vi "Send Alternative Long Execution Method.vi"(7 "Async Message Settings":T1={"Message Priority (Normal)"=enum."Normal", "Async Call Method (Call and Collect)"=enum."Call and Collect", "VI Refnum Lifetime (Destroy on Actor Exit)"=enum."Destroy on Actor Exit", "Report Errors (T)"=TRUE, "Caller Enqueuer"=refnum, "Completion Notification Msg"=refnum}, 8 "error in (no error)":errorcluster, 11 "Message Enqueuer in":refnum<class "Message Enqueuer.lvclass">) -> (0 "error out":errorcluster, 2 "GUID":string, 3 "Message Enqueuer out":refnum<class "Message Enqueuer.lvclass">)   [LabVIEW 2023, in "Async Methods Actor Example.lvlib" / "Alternative Long Execution Method Msg.lvclass"]
doc: "Sends the <b>Async Methods Actor Example.lvlib:Alternative Long Execution Method Msg.lvclass</b> Async Message.\n\nThis message will call <b>Alternative Long Execution Method.vi</b> on the <b>Async Methods Actor Example.lvlib:Async Methods Actor Example.lvclass</b> Async Method Actor.\n\n<b>Alternative Long Execution Method.vi Description</b>"
uses:
  Alternative Long Execution Method Msg.lvclass
  Alternative Long Execution Method Msg.lvclass/Alternative Long Execution Method Msg.ctl
  Async Methods Actor/Async Methods Actor Messages/Async Message/Async Message.lvclass
  <vilib>/ActorFramework/Message Enqueuer/Message Priority.ctl
  <vilib>/ActorFramework/Message Enqueuer/Message Enqueuer.lvclass
  Async Methods Actor/Async Methods Actor/Async Call Method.ctl
  Async Methods Actor/Async Methods Actor/Async Methods Actor.lvclass
  Async Methods Actor/Async Methods Actor/VI Refnum Lifetime.ctl
  Async Methods Actor/Async Methods Actor Messages/Completion Notification Msg/Completion Notification Msg.lvclass
  Async Methods Actor/Async Methods Actor Messages/Async Message/Async Message Settings.ctl
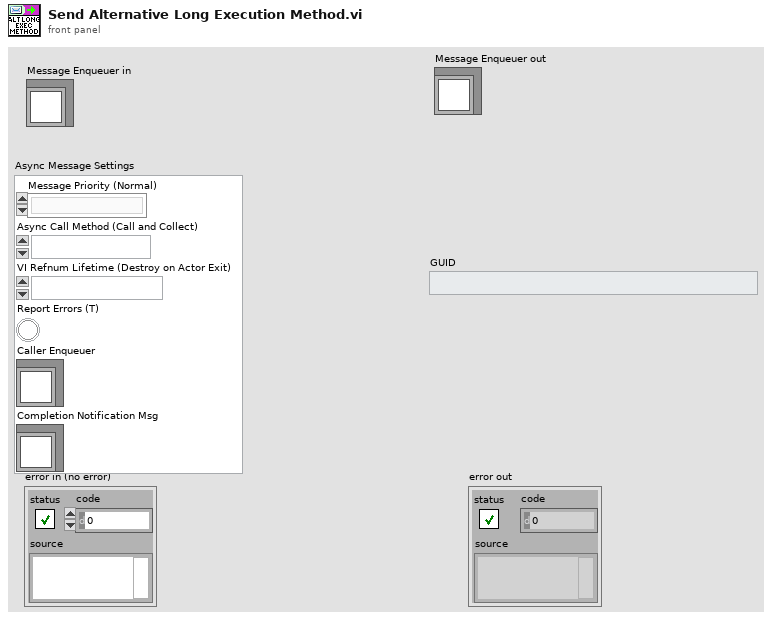
[diagram p1: front panel]
types:
  T1 = typedef "Async Methods Actor.lvlib/Async Message.lvclass/Async Message Settings.ctl" = cluster{"Message Priority (Normal)":T2, "Async Call Method (Call and Collect)":T3, "VI Refnum Lifetime (Destroy on Actor Exit)":T4, "Report Errors (T)":bool, "Caller Enqueuer":refnum<class "Message Enqueuer.lvclass">, "Completion Notification Msg":refnum<class "Completion Notification Msg.lvclass">}
  T2 = typedef "Actor Framework.lvlib/Message Enqueuer.lvclass/Message Priority.ctl" = enum16{"Low", "Normal", "High"}
  T3 = typedef "Async Methods Actor.lvlib/Async Methods Actor.lvclass/Async Call Method.ctl" = enum16{"Call and Collect", "Call and Forget"}
  T4 = typedef "Async Methods Actor.lvlib/Async Methods Actor.lvclass/VI Refnum Lifetime.ctl" = enum16{"Destroy on Exit", "Destroy on Actor Exit", "Destroy on Application Exit"}
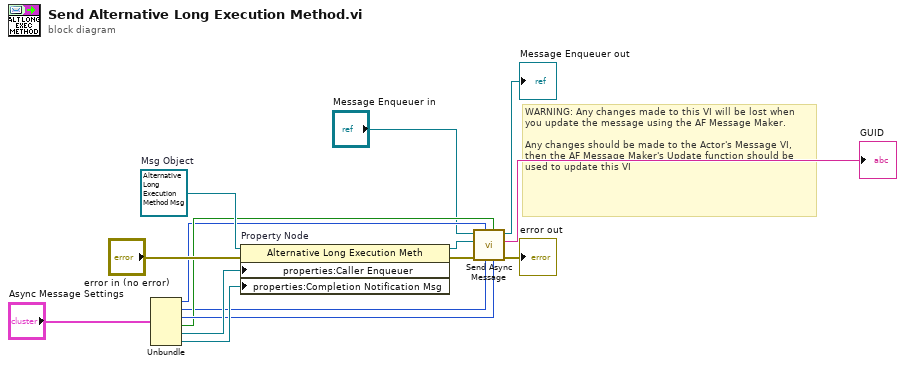
[diagram p0: block diagram]
diagram:
  w13 = refnum<class "Alternative Long Execution Method Msg.lvclass"> refnum  # Msg Object
  # "WARNING: Any changes made to this VI will be lost when you update the message using the AF Message Maker.\n\nAny changes should be made to the Actor's Message VI, then the AF Message Maker's Update function should be used to update this VI"
  n1 = Unbundle "Unbundle"("Async Message Settings") -> ("Message Priority (Normal)"=w4:T2, "Async Call Method (Call and Collect)"=w5:T3, "VI Refnum Lifetime (Destroy on Actor Exit)"=w7:T4, "Report Errors (T)"=w6:bool, "Caller Enqueuer"=w12:refnum<class "Message Enqueuer.lvclass">, "Completion Notification Msg"=w11:refnum<class "Completion Notification Msg.lvclass">)
  n2 = property on="Property Node" class="Alternative Long Execution Meth"(reference=w13, error in="error in (no error)", "properties:Caller Enqueuer"=w12, "properties:Completion Notification Msg"=w11) -> (reference out=w2:refnum<class "Alternative Long Execution Method Msg.lvclass">, error out=w3:errorcluster)
  n3 = call "Send Async Message.vi"("VI Refnum Lifetime (Destroy on Actor Exit)"=w7, "Report Errors (T)"=w6, "Async Call Method (Call and Collect)"=w5, "Message Priority (Normal)"=w4, "error in (no error)"=w3, "Concrete Async Message"=w2, "Message Enqueuer"="Message Enqueuer in") -> ("error out"=→"error out":errorcluster, "GUID"=→"GUID":string, "Message Enqueuer out"=→"Message Enqueuer out":refnum<class "Message Enqueuer.lvclass">)  [unwired: 2 in]
